vi "1_CreateClient.vi"(8 "error in (no error)":errorcluster caption="错误输入（无错误）", 10 "Create":T1={"address"="localhost", "port"=1883, "UserName"="", "Pwd"=""}, 11 "MQTT_Client_Actor 输入":refnum<class "MQTT_Client_Actor.lvclass">) -> (0 "error out":errorcluster caption="错误输出", 3 "MQTT_Client_Actor 输出":refnum<class "MQTT_Client_Actor.lvclass">)   [LabVIEW 2018, in "MQTT_Client_Actor.lvlib" / "MQTT_Client_Actor.lvclass"]
uses:
  MQTT_Client_Actor.lvclass
  CreateClient.ctl
  MQTT_Client_Actor.lvclass/MQTT_Client_Actor.ctl
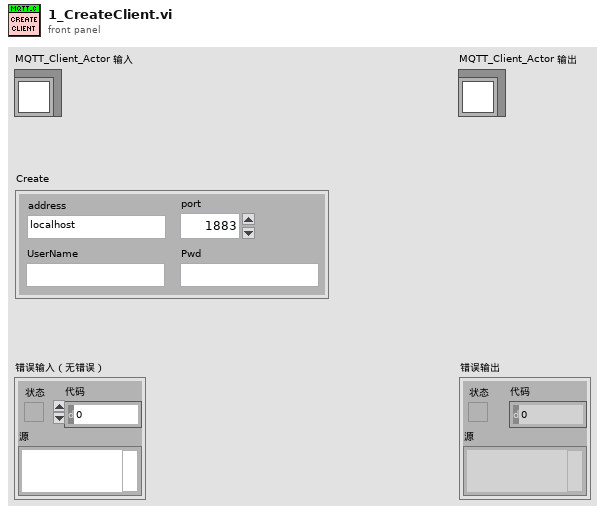
[diagram p1: front panel]
types:
  T1 = typedef "MQTT_Client_Actor.lvlib/MQTT_Client_Actor.lvclass/CreateClient.ctl" = cluster{"address":string, "port":u16, "UserName":string, "Pwd":string}
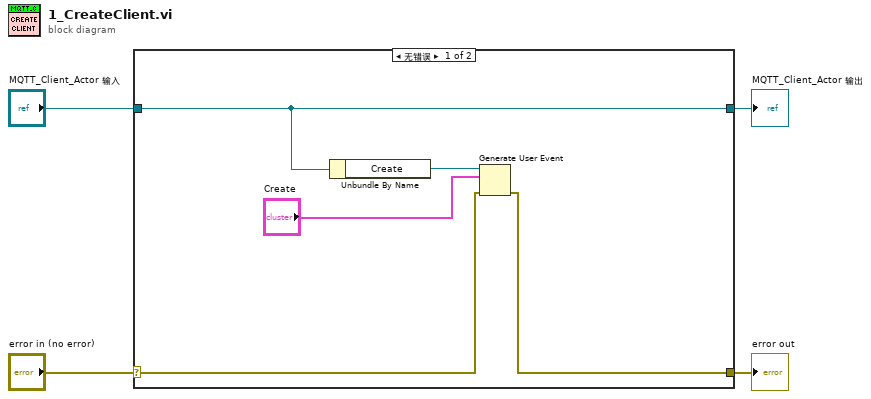
[diagram p0: block diagram]
diagram:
  n1 = case shown="无错误" "error in (no error)" {
    selector: "error in (no error)" -> [w8 w11]
    tunnel: [w7 w11] -> w3
    tunnel: [w9 w10] -> w1
    tunnel: "MQTT_Client_Actor 输入" -> [w9 w10]
    frame No Error {
      n2 = Unbundle By Name(w9) -> ("Create"=w6:refnum<user-event>)
      n3 = Generate User Event(user event=w6, event data cluster="Create", error in=w8) -> (error out=w7:errorcluster)  [unwired: 1 in, 1 out]
    }
    frame Error {
    }
  }
  "error out" <- w3
  "MQTT_Client_Actor 输出" <- w1
